vi "Options.vi"(8 "error in (no error)":errorcluster, 9 "Arriving from":enum16{"North", "South", "East", "West"}(ring), 10 "Cluster":cluster{"row":i32, "col":i32}, 11 "Maze In":refnum<class "Maze.lvclass">) -> (0 "error out":errorcluster, 2 "Possible Steps":T1(array[cluster]), 3 "Maze Out":refnum<class "Maze.lvclass">)   [LabVIEW 2021, in "Maze.lvclass"]
uses:
  Maze.lvclass
  Maze.lvclass/Maze.ctl
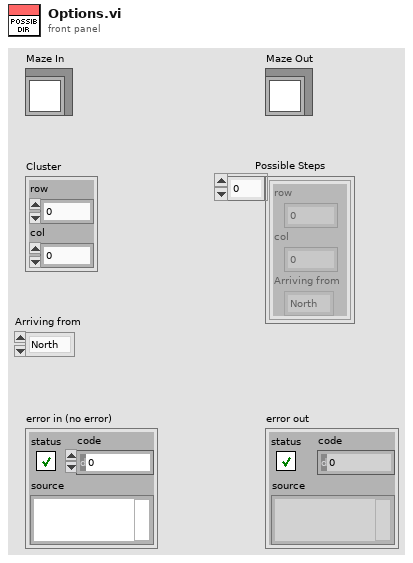
[diagram p1: front panel]
types:
  T1 = cluster{"row":i32, "col":i32, "Arriving from":enum16{"North", "South", "East", "West"}}[]
  T2 = cluster{"row":i32, "col":i32, "Arriving from":enum16{"North", "South", "East", "West"}}
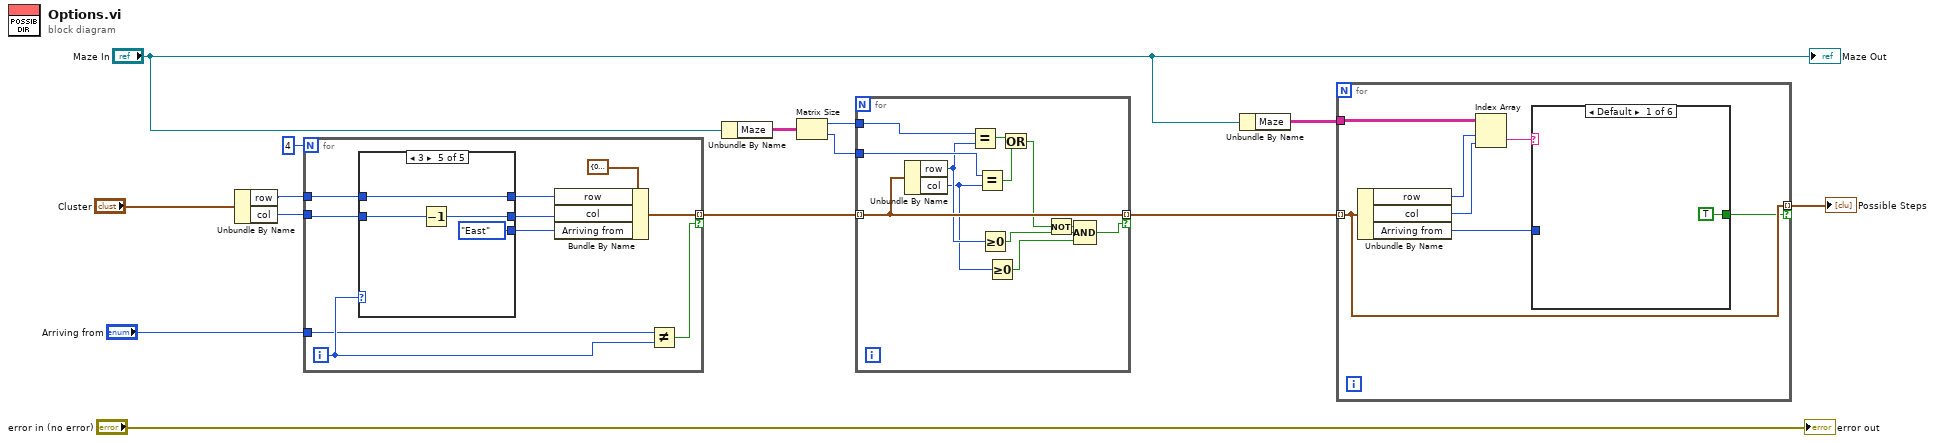
[diagram p0: block diagram]
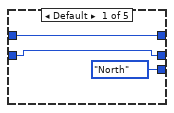
[diagram p2: hidden frame]
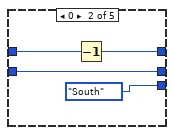
[diagram p3: hidden frame]
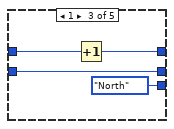
[diagram p4: hidden frame]
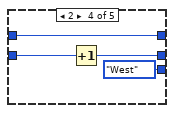
[diagram p5: hidden frame]
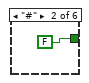
[diagram p6: hidden frame]
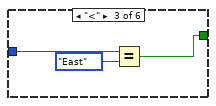
[diagram p7: hidden frame]
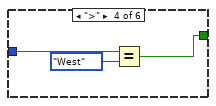
[diagram p8: hidden frame]
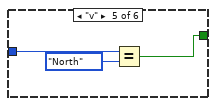
[diagram p9: hidden frame]
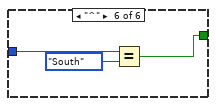
[diagram p10: hidden frame]
diagram:
  n1 = Unbundle By Name("Cluster") -> ("row"=w12:i32, "col"=w11:i32)
  n2 = for {
    N: 4 -> [_]
    tunnel: w12 -> [w24]
    tunnel: w11 -> [w23]
    tunnel: [w19] -> w5 mode=indexing if=w16
    tunnel: "Arriving from" -> [w17]
    i -> [w18]
    n3 = case shown="3" w18 {
      tunnel: w24 -> [w27 w31 w35 w39 w43]
      tunnel: [w26 w30 w34 w37 w41] -> w20
      tunnel: w23 -> [w26 w30 w34 w38 w42]
      tunnel: [w27 w29 w33 w39 w43] -> w21
      tunnel: [enum16{"North", "South", "East", "West"}."North" ("Arriving from") enum16{"North", "South", "East", "West"}."South" ("Arriving from") enum16{"North", "South", "East", "West"}."North" ("Arriving from") enum16{"North", "South", "East", "West"}."West" ("Arriving from") enum16{"North", "South", "East", "West"}."East" ("Arriving from")] -> w15
      frame Default {
      }
      frame 0 {
        n4 = Decrement(x=w31) -> (x-1=w29:i32)
      }
      frame 1 {
        n5 = Increment(x=w35) -> (x+1=w33:i32)
      }
      frame 2 {
        n6 = Increment(x=w38) -> (x+1=w37:i32)
      }
      frame 3 {
        n7 = Decrement(x=w42) -> (x-1=w41:i32)
      }
    }
    n8 = Bundle By Name(cluster=T2 {"row"=0, "col"=0, "Arriving from"=enum."North"} ("Cluster"), "row"=w21, "col"=w20, "Arriving from"=w15) -> (w19:T2)
    n9 = Not Equal?(x=w17, y=w18) -> (x != y?=w16:bool)
  }
  n10 = Unbundle By Name("Maze In") -> ("Maze"=w7:string[][])
  n11 = Matrix Size(0:w7) -> (1:w4:i32, 2:w3:i32)
  n12 = for {
    tunnel: w5 -> [w55] mode=indexing
    tunnel: [w55] -> w1 mode=indexing if=w46
    tunnel: w4 -> [w54]
    tunnel: w3 -> [w53]
    n13 = Unbundle By Name(w55) -> ("row"=w48:i32, "col"=w47:i32)
    n14 = Equal?(x=w54, y=w48) -> (x = y?=w52:bool)
    n15 = Equal?(x=w53, y=w47) -> (x = y?=w51:bool)
    n16 = Greater Or Equal To 0?(x=w48) -> (x >= 0?=w45:bool)
    n17 = Greater Or Equal To 0?(x=w47) -> (x >= 0?=w44:bool)
    n18 = Or(x=w52, y=w51) -> (x .or. y?=w50:bool)
    n19 = Not(x=w50) -> (.not. x?=w49:bool)
    n20 = Compound Arithmetic op=AND(w49, w45, w44) -> (w46:bool)
  }
  n21 = Unbundle By Name("Maze In") -> ("Maze"=w6:string[][])
  n22 = for {
    tunnel: w6 -> [w62]
    tunnel: w1 -> [w57] mode=indexing
    tunnel: [w57] -> w8 mode=indexing if=w56
    n23 = Unbundle By Name(w57) -> ("row"=w61:i32, "col"=w60:i32, "Arriving from"=w58:enum16{"North", "South", "East", "West"})
    n24 = Index Array(array=w62, index (row)=w61, index (col)=w60) -> (element=w59:string)
    n25 = case shown="Default" w59 {
      tunnel: w58 -> [_ _ w67 w70 w73 w76]
      tunnel: [TRUE FALSE w65 w68 w71 w74] -> w56
      frame Default {
      }
      frame "#" {
      }
      frame "<" {
        n26 = Equal?(x=w67, y=enum16{"North", "South", "East", "West"}."East") -> (x = y?=w65:bool)
      }
      frame ">" {
        n27 = Equal?(x=w70, y=enum16{"North", "South", "East", "West"}."West") -> (x = y?=w68:bool)
      }
      frame "v" {
        n28 = Equal?(x=w73, y=enum16{"North", "South", "East", "West"}."North") -> (x = y?=w71:bool)
      }
      frame "^" {
        n29 = Equal?(x=w76, y=enum16{"North", "South", "East", "West"}."South") -> (x = y?=w74:bool)
      }
    }
  }
  "Possible Steps" <- w8
  "error out" <- "error in (no error)"
  "Maze Out" <- "Maze In"
